vi "Test Default Audio Device Playback.vi"(8 "error in (no error)":errorcluster) -> (0 "error out":errorcluster, 3 "Pass?":bool)   [LabVIEW 2020]
uses:
  G-Audio/Controls/Backends.ctl
  G-Audio/Controls/Audio Device Info.ctl
  G-Audio/Controls/Audio Device Type.ctl
  G-Audio/Audio Files/Polymorphic VIs/Quick Load Audio File (Path).vi
  678bb3a3-ab52-4f1b-8279-67e7041d0764.vi
  G-Audio/Private/Path To UTF-8 String.vi
  G-Audio/Audio Files/Private/Quick Load Audio File (Core).vi
  G-Audio/Private/Result To Error.vi
  678bb3a3-ab52-4f1b-8279-67e7041d0764.vi/4dfb5711-8d81-45a3-b3db-a84d40650863.vi
  678bb3a3-ab52-4f1b-8279-67e7041d0764.vi/c8869513-30c6-44f2-a2d3-73232fe63870.vi
  678bb3a3-ab52-4f1b-8279-67e7041d0764.vi/4dfb5711-8d81-45a3-b3db-a84d40650863.vi/4b7b629c-2e91-4160-9820-a26af8f6e677.vi
  678bb3a3-ab52-4f1b-8279-67e7041d0764.vi/c8869513-30c6-44f2-a2d3-73232fe63870.vi/4b7b629c-2e91-4160-9820-a26af8f6e677.vi
  <vilib>/Utility/error.llb/Error Cluster From Error Code.vi
  G-Audio/Private/Copy Data.vi
  <vilib>/Utility/Data Type/Get Numeric Information.vi
  G-Audio/G-Audio.lvlib
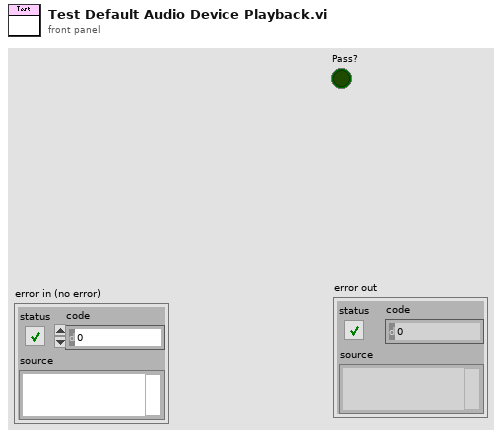
[diagram p1: front panel]
types:
  T1 = typedef "G-Audio.lvlib/Backends.ctl" = enum16{"WASAPI", "DirectSound", "WinMM", "Core Audio", "sndio", "audio(4)", "OSS", "PulseAudio", "ALSA", "JACK", "AAudio", "OpenSL|ES", "Web Audio", "Custom", "Null", "Default"}
  T2 = typedef "G-Audio.lvlib/Audio Device Info.ctl" = cluster{"Name":string, "ID":u8[], "Device Type":T3}
  T3 = typedef "G-Audio.lvlib/Audio Device Type.ctl" = enum16{"(None)", "Playback", "Capture", "Duplex", "Loopback"}
  T4 = typedef "G-Audio.lvlib/Audio Device Refnum.ctl" = refnum<file>
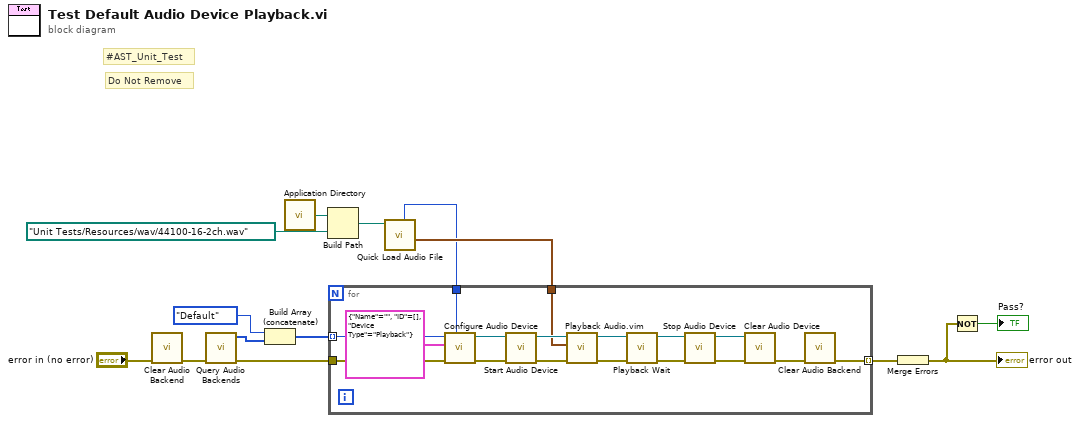
[diagram p0: block diagram]
diagram:
  # "Do Not Remove"
  # "#AST_Unit_Test"
  n1 = call "Clear Audio Backend.vi"("error in (no error)"="error in (no error)") -> ("error out"=w1:errorcluster)  [unwired: 10 in]
  n2 = call "Query Audio Backends.vi"("error in (no error)"=w1) -> ("error out"=w14:errorcluster, "Backends"=w13:T1[])  [unwired: 9 in]
  n3 = Build Array (concatenate)(Backends."Default" ("Backends"), w13) -> (w11:T1[])
  n4 = call <vilib>:"Application Directory.vi"() -> ("Application Directory"=w10:path)
  n5 = Build Path(base path=w10, name or relative path=path "Unit Tests/Resources/wav/44100-16-2ch.wav" ("Path")) -> (appended path=w8:path)
  n6 = call-poly "Quick Load Audio File.vi"("Path"=w8) -> ("data"=w7:waveform(i16)[], "PCM Frame Length"=w6:u64)  [unwired: 5 in, 4 out]
  n7 = for {
    tunnel: w14 -> [w24]
    tunnel: w11 -> [w23] mode=indexing
    tunnel: w7 -> [w21]
    tunnel: w6 -> [w20]
    tunnel: [w15] -> w5 mode=indexing
    n8 = call "Configure Audio Device.vi"("Buffer Size (4096)"=w20, "error in (no error)"=w24, "Audio Device"=T2 {"Name"="", "ID"=[], "Device Type"=enum."Playback"}, "Backend (Default)"=w23) -> ("error out"=w30:errorcluster, "Audio Device Refnum"=w31:T4)  [unwired: 6 in]
    n9 = call "Start Audio Device.vi"("error in (no error)"=w30, "Audio Device Refnum In"=w31) -> ("error out"=w28:errorcluster, "Audio Device Refnum Out"=w29:T4)  [unwired: 8 in]
    n10 = call "Playback Audio.vim"("error in (no error)"=w28, "Audio Data"=w21, "Audio Device Refnum In"=w29) -> ("error out"=w17:errorcluster, "Audio Device Refnum Out"=w19:T4)  [unwired: 7 in]
    n11 = call "Playback Wait.vi"("error in (no error)"=w17, "Audio Device Refnum In"=w19) -> ("error out"=w16:errorcluster, "Audio Device Refnum Out"=w18:T4)  [unwired: 8 in]
    n12 = call "Stop Audio Device.vi"("error in (no error)"=w16, "Audio Device Refnum In"=w18) -> ("error out"=w26:errorcluster, "Audio Device Refnum Out"=w25:T4)  [unwired: 8 in]
    n13 = call "Clear Audio Device.vi"("error in (no error)"=w26, "Audio Device Refnum In"=w25) -> ("error out"=w27:errorcluster)  [unwired: 9 in]
    n14 = call "Clear Audio Backend.vi"("error in (no error)"=w27) -> ("error out"=w15:errorcluster)  [unwired: 10 in]
  }
  n15 = Merge Errors(w5) -> (w4:errorcluster)
  "error out" <- w4
  n16 = Not(x=w4) -> (.not. x?=→"Pass?":bool)
